vi "JSON_parser.vi"() -> ()   [LabVIEW 2020]
uses:
  <vilib>/LVH/i3 JSON/JSON Parsing/Get Object Parameter Files/Get Object Parameter - String.vi
  <vilib>/LVH/i3 JSON/JSON Parsing/Get Object Parameter Files/Get Object Parameter - Object.vi
  <vilib>/LVH/i3 JSON/JSON Parsing/Get Object Parameter Files/Get Object Parameter - Numeric.vi
  <vilib>/LVH/i3 JSON/i3-json.lvlib
panel:
  out "Miasto":string
  out "Temperatura":dbl
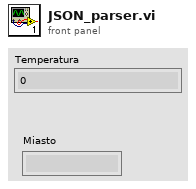
[diagram p1: front panel]
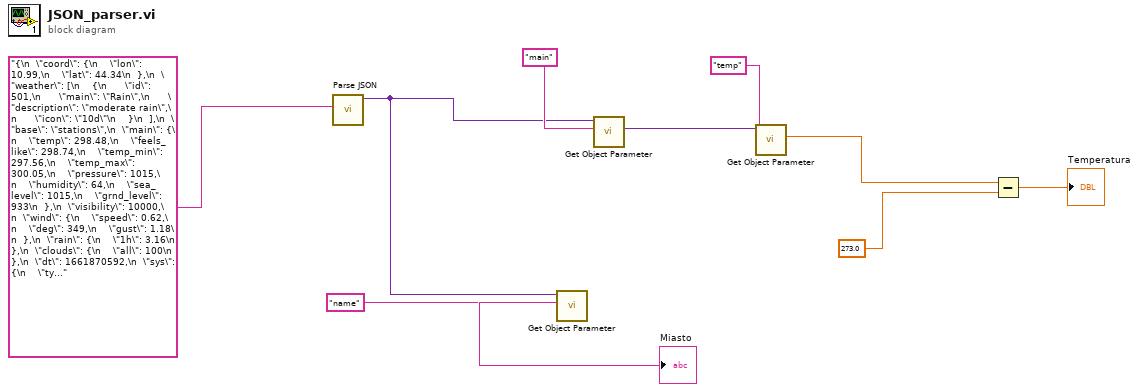
[diagram p0: block diagram]
diagram:
  n1 = call <vilib>:"Parse JSON.vi"("JSON String"="{\n  \"coord\": {\n    \"lon\": 10.99,\n    \"lat\": 44.34\n  },\n  \"weather\": [\n    {\n      \"id\": 501,\n      \"main\": \"Rain\",\n      \"description\": \"moderate rain\",\n      \"icon\": \"10d\"\n    }\n  ],\n  \"base\": \"stations\",\n  \"main\": {\n    \"temp\": 298.48,\n    \"feels_like\": 298.74,\n    \"temp_min\": 297.56,\n    \"temp_max\": 300.05,\n    \"pressure\": 1015,\n    \"humidity\": 64,\n    \"sea_level\": 1015,\n    \"grnd_level\": 933\n  },\n  \"visibility\": 10000,\n  \"wind\": {\n    \"speed\": 0.62,\n    \"deg\": 349,\n    \"gust\": 1.18\n  },\n  \"rain\": {\n    \"1h\": 3.16\n  },\n  \"clouds\": {\n    \"all\": 100\n  },\n  \"dt\": 1661870592,\n  \"sys\": {\n    \"type\": 2,\n    \"id\": 2075663,\n    \"country\": \"IT\",\n    \"sunrise\": 1661834187,\n    \"sunset\": 1661882248\n  },\n  \"timezone\": 7200,\n  \"id\": 3163858,\n  \"name\": \"Zocca\",\n  \"cod\": 200\n}                        ") -> ("JSON Tree"=w1:variant)  [unwired: 7 in, 3 out]
  n2 = call-poly <vilib>:"Get Object Parameter.vi"("Parameter Name"="name", "JSON Tree In (JSON Object)"=w1) -> ("String Value"=→"Miasto":string)  [unwired: 6 in, 3 out]
  n3 = call-poly <vilib>:"Get Object Parameter.vi"("Parameter Name"="main", "JSON Tree In (JSON Object)"=w1) -> ("JSON Object"=w8:variant)  [unwired: 6 in, 3 out]
  n4 = call-poly <vilib>:"Get Object Parameter.vi"("Parameter Name"="temp", "JSON Tree In (JSON Object)"=w8) -> ("Double Value"=w7:dbl)  [unwired: 6 in, 3 out]
  n5 = Subtract(x=w7, y=273.0) -> (x-y=→"Temperatura":dbl)
